vi "Generate VI HTML.vi"(7 "Generation options":T1={"Minify?"=FALSE, "Disabled Tabs"=[], "Default Tab"=enum."FP"}, 8 "error in":errorcluster, 10 "Output path":path, 11 "VI Path":path) -> (0 "error out":errorcluster)   [LabVIEW 2019]
uses:
  Typedefs/Generation options.ctl
  Typedefs/Tab.ctl
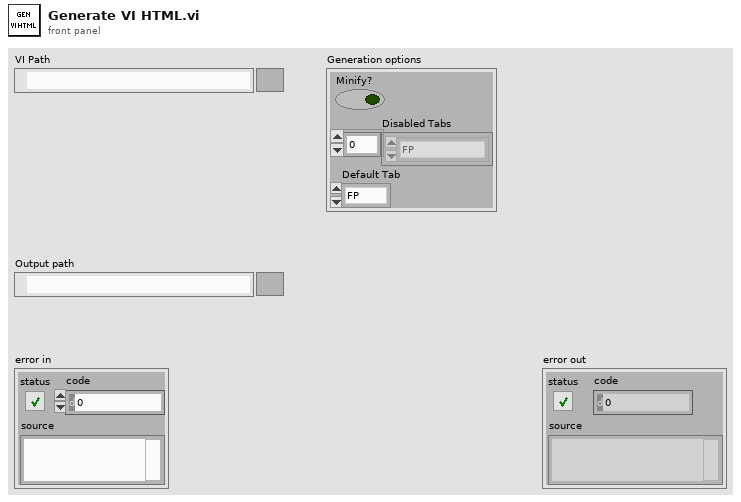
[diagram p1: front panel]
types:
  T1 = typedef "Generation options.ctl" = cluster{"Minify?":bool, "Disabled Tabs":T2[], "Default Tab":T2}
  T2 = typedef "Tab.ctl" = enum16{"Info", "FP", "BD"}
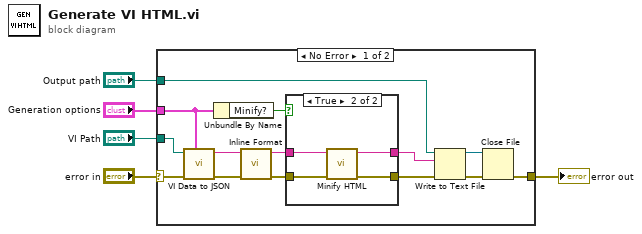
[diagram p0: block diagram]
diagram:
  n1 = case shown="No Error" "error in" {
    selector: "error in" -> [w7 w26]
    tunnel: [w17 w26] -> w5
    tunnel: "Output path" -> [w16 _]
    tunnel: "VI Path" -> [w6 _]
    tunnel: "Generation options" -> [w8 _]
    frame No Error {
      n2 = call "VI Data to JSON.vi"("Generation options"=w8, "error in"=w7, "VI Path"=w6) -> ("error out"=w15:errorcluster, "JSON string"=w14:string)  [unwired: 7 in]
      n3 = Unbundle By Name(w8) -> ("Minify?"=w9:bool)
      n4 = call "Inline Format.vi"("error in"=w15, "VI JSON"=w14) -> ("error out"=w13:errorcluster, "Inlined HTML"=w11:string)  [unwired: 8 in]
      n5 = case shown="True" w9 {
        tunnel: w13 -> [w20 w25]
        tunnel: [w20 w24] -> w12
        tunnel: w11 -> [w21 w23]
        tunnel: [w21 w22] -> w10
        frame False {
        }
        frame True {
          n6 = call "Minify HTML.vi"("error in (no error)"=w25, "HTML in"=w23) -> ("error out"=w24:errorcluster, "Minified HTML"=w22:string)  [unwired: 8 in]
        }
      }
      n7 = Write to Text File(file (use dialog)=w16, text=w10, error in=w12) -> (refnum out=w19:refnum<file>, error out=w18:errorcluster)  [unwired: 1 in, 1 out]
      n8 = Close File(refnum=w19, error in=w18) -> (error out=w17:errorcluster)  [unwired: 1 out]
    }
    frame Error {
    }
  }
  "error out" <- w5
